vi "Init.vi"(8 "error in (no error)":errorcluster, 11 "Stream in":refnum<class "Stream.lvclass">) -> (0 "error out":errorcluster, 3 "Stream out":refnum<class "Stream.lvclass">)   [LabVIEW 2018, in "Stream.lvclass"]
uses:
  Stream.lvclass
  Stream.lvclass/Stream.ctl
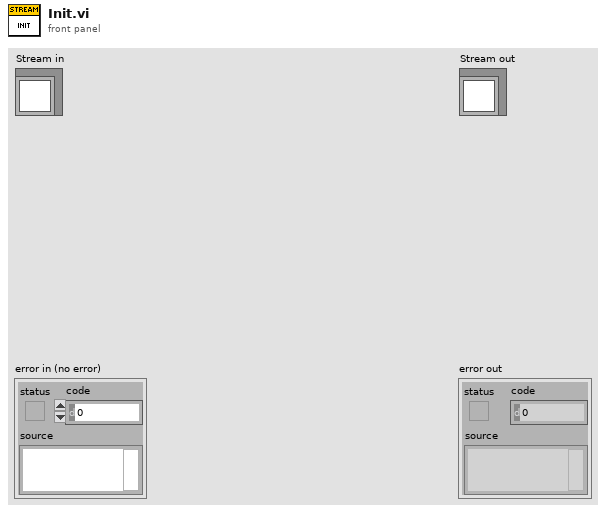
[diagram p1: front panel]
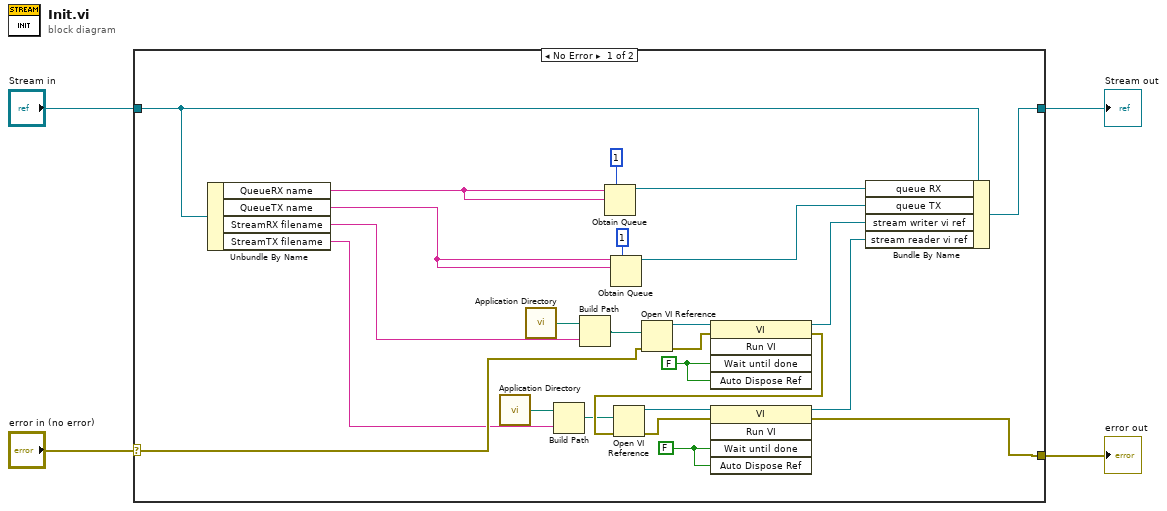
[diagram p0: block diagram]
diagram:
  n1 = case shown="No Error" "error in (no error)" {
    selector: "error in (no error)" -> [w12 w31]
    tunnel: [w11 w31] -> w3
    tunnel: [w5 w30] -> w1
    tunnel: "Stream in" -> [w6 w30]
    frame No Error {
      w26 = FALSE ("Wait Until Done")
      w21 = FALSE ("Wait Until Done")
      n2 = Unbundle By Name(w6) -> ("QueueRX name"=w10:string, "QueueTX name"=w9:string, "StreamRX filename"=w8:string, "StreamTX filename"=w7:string)
      n3 = call <vilib>:"Application Directory.vi"() -> ("Application Directory"=w23:path)
      n4 = call <vilib>:"Application Directory.vi"() -> ("Application Directory"=w27:path)
      n5 = Build Path(base path=w23, name or relative path=w7) -> (appended path=w22:path)
      n6 = Build Path(base path=w27, name or relative path=w8) -> (appended path=w28:path)
      n7 = Obtain Queue(max queue size (-1, unlimited)=1, name (unnamed)=w10, element data type=w10) -> (queue out=w13:refnum<queue>)  [unwired: 2 in, 2 out]
      n8 = Obtain Queue(max queue size (-1, unlimited)=1, name (unnamed)=w9, element data type=w9) -> (queue out=w14:refnum<queue>)  [unwired: 2 in, 2 out]
      n9 = Open VI Reference(vi path=w28, error in (no error)=w12) -> (vi reference=w20:refnum<vi>, error out=w19:errorcluster)  [unwired: 4 in]
      n10 = invoke class="VI" method="Run VI"(reference=w20, error in=w19, "Wait until done"=w21, "Auto Dispose Ref"=w21) -> (reference out=w18:refnum<vi>, error out=w29:errorcluster)  [unwired: 1 in, 3 out]
      n11 = Open VI Reference(vi path=w22, error in (no error)=w29) -> (vi reference=w24:refnum<vi>, error out=w25:errorcluster)  [unwired: 4 in]
      n12 = invoke class="VI" method="Run VI"(reference=w24, error in=w25, "Wait until done"=w26, "Auto Dispose Ref"=w26) -> (reference out=w17:refnum<vi>, error out=w11:errorcluster)  [unwired: 1 in, 3 out]
      n13 = Bundle By Name(cluster=w6, "queue RX"=w13, "queue TX"=w14, "stream writer vi ref"=w18, "stream reader vi ref"=w17) -> (w5:refnum<class "Stream.lvclass">)
    }
    frame Error {
    }
  }
  "error out" <- w3
  "Stream out" <- w1
